vi "AO Acquisition Setup.vi"(11 "Analog Output Data":T1) -> (0 "error out":errorcluster, 3 "Refnum out":refnum<k21>)   [LabVIEW 2021]
doc: "This VI receives the cluster data necessary to setup and start the DAQmx analog output data acquisition."
uses:
  <vilib>/DAQmx/create/channels.llb/DAQmx Create Channel (AO-Voltage-Basic).vi
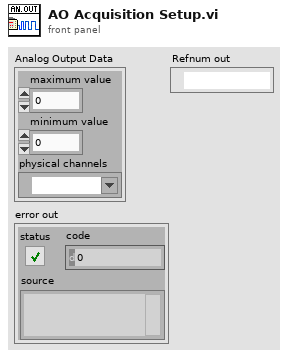
[diagram p1: front panel]
types:
  T1 = cluster{"maximum value":dbl, "minimum value":dbl, "physical channels":tag}
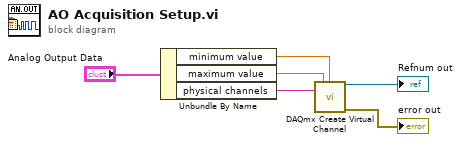
[diagram p0: block diagram]
diagram:
  n1 = Unbundle By Name("Analog Output Data") -> ("minimum value"=w4:dbl, "maximum value"=w5:dbl, "physical channels"=w6:tag)
  n2 = call-poly <vilib>:"DAQmx Create Virtual Channel.vi"("maximum value"=w5, "minimum value"=w4, "physical channels"=w6) -> ("task out"=→"Refnum out":refnum<k21>, "error out"=→"error out":errorcluster)  [unwired: 11 in]
